vi "DevB.API Test.vi"() -> ()   [LabVIEW 2018]
panel:
  out "Connected":bool
  in  "Port":refnum<visa-resource-name>
  out "error out":errorcluster
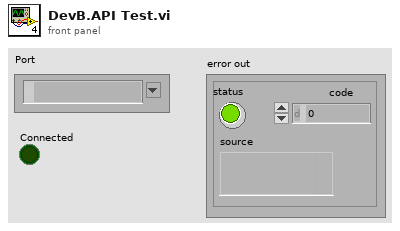
[diagram p1: front panel]
types:
  T1 = typedef "DevB.Session.ctl" = cluster{"DevBoard Ref":refnum<visa-resource-name>}
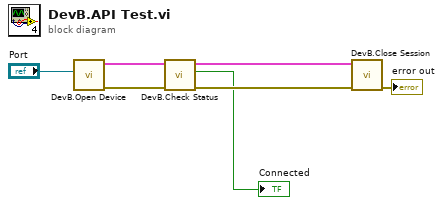
[diagram p0: block diagram]
diagram:
  n1 = call "DevB.Open Device.vi"("Port"="Port") -> ("error out"=w4:errorcluster, "DevB Session out"=w5:T1)  [unwired: 9 in]
  n2 = call "DevB.Check Status.vi"("error in (no error)"=w4, "DevB Session in"=w5) -> ("error out"=w2:errorcluster, "Connected"=→"Connected":bool, "DevB Session out"=w3:T1)  [unwired: 7 in]
  n3 = call "DevB.Close Session.vi"("error in (no error)"=w2, "DevB Session"=w3) -> ("error out"=→"error out":errorcluster)  [unwired: 9 in]
